vi "get channels.vi"(11 "user tag bus module configuration In":refnum<class "TEST CONFIGURATION.lvclass">) -> (2 "channels":refnum<class "TBM channel.lvclass">[](array[class]), 3 "user tag bus module configuration Out":refnum<class "TEST CONFIGURATION.lvclass">)   [LabVIEW 2013, in "configuration tests.lvlib" / "TEST CONFIGURATION.lvclass"]
uses:
  TEST CONFIGURATION.lvclass
  <vilib>/NI/Tag Bus Module Framework/channel/TBM channel.lvclass
  TEST CONFIGURATION.lvclass/TEST CONFIGURATION.ctl
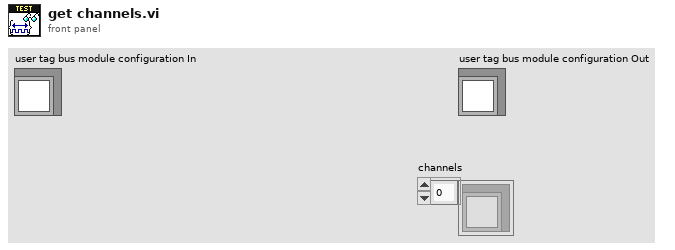
[diagram p1: front panel]
types:
  T1 = typedef "configuration tests.lvlib/TEST CONFIGURATION.lvclass/state module configuration.ctl" = cluster{"fixed input":refnum<class "TBM channel.lvclass">, "fixed output":refnum<class "TBM channel.lvclass">, "initial state":u8}
  T2 = typedef "configuration tests.lvlib/TEST CONFIGURATION.lvclass/control module configuration.ctl" = cluster{"name":string, "setpoint":refnum<class "TBM channel.lvclass">, "process variable":refnum<class "TBM channel.lvclass">, "output":refnum<class "TBM channel.lvclass">, "gains":T3, "output range":cluster{"output high":dbl, "output low":dbl}}
  T3 = typedef "configuration tests.lvlib/TEST CONFIGURATION.lvclass/gains.ctl" = cluster{"Kp":dbl, "Ki":dbl, "Kd":dbl}
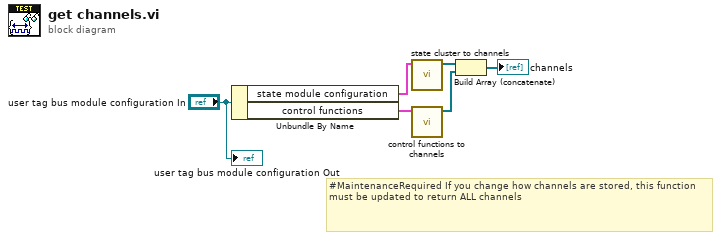
[diagram p0: block diagram]
diagram:
  # "#MaintenanceRequired If you change how channels are stored, this function must be updated to return ALL channels"
  n1 = Unbundle By Name("user tag bus module configuration In") -> ("state module configuration"=w5:T1, "control functions"=w4:T2[])
  n2 = call "state cluster to channels.vi"("state module configuration"=w5) -> ("channels"=w1:refnum<class "TBM channel.lvclass">[])  [unwired: 10 in]
  n3 = call "control functions to channels.vi"("control functions"=w4) -> ("channels"=w3:refnum<class "TBM channel.lvclass">[])  [unwired: 10 in]
  n4 = Build Array (concatenate)(w1, w3) -> (→"channels":refnum<class "TBM channel.lvclass">[])
  "user tag bus module configuration Out" <- "user tag bus module configuration In"
